vi "scaled pythagorean.vi"(2 "c":dbl, 3 "b":dbl, 4 "a":dbl) -> (0 "b":dbl, 1 "a":dbl)   [LabVIEW 2009]
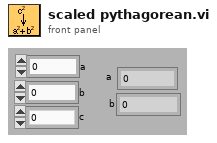
[diagram p1: front panel]
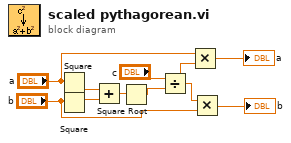
[diagram p0: block diagram]
diagram:
  n1 = Square(x="a") -> (x^2=w10:dbl)
  n2 = Square(x="b") -> (x^2=w9:dbl)
  n3 = Add(x=w10, y=w9) -> (x+y=w8:dbl)
  n4 = Square Root(x=w8) -> (sqrt(x)=w6:dbl)
  n5 = Divide(x="c", y=w6) -> (x/y=w5:dbl)
  n6 = Multiply(x="a", y=w5) -> (x*y=→"a":dbl)
  n7 = Multiply(x=w5, y="b") -> (x*y=→"b":dbl)
